vi "FindAllSupportedModules.vi"(11 "Device Model":T1) -> (2 "All Supported Modules":string[](array[string]), 3 "Number of Supported Modules":i32)   [LabVIEW 2015]
uses:
  <vilib>/addons/InsightCM/MessageBus/Base/controls/Device.ctl
  <vilib>/addons/InsightCM/MessageBus/Base/controls/KeyValuePair.ctl
  <vilib>/addons/InsightCM/MessageBus/Base/controls/DataGroup.ctl
  <vilib>/addons/InsightCM/MessageBus/Base/controls/OperatingState.ctl
  <vilib>/addons/InsightCM/MessageBus/Base/controls/Trigger.ctl
  <vilib>/addons/InsightCM/MessageBus/Base/controls/Condition.ctl
  <vilib>/addons/InsightCM/Utilities/DeviceModelHelpers/DeviceModelHelpers.lvlib
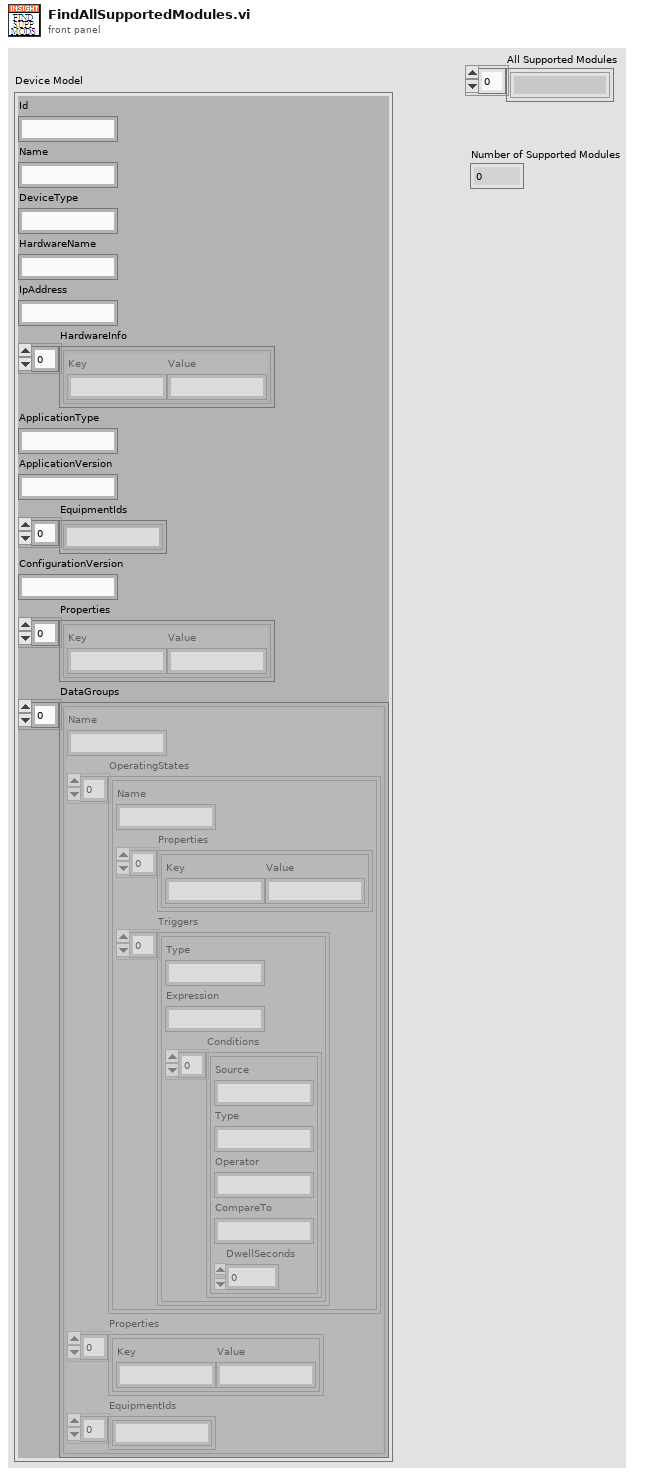
[diagram p1: front panel]
types:
  T1 = typedef "Device.ctl" = cluster{"Id":string, "Name":string, "DeviceType":string, "HardwareName":string, "IpAddress":string, "HardwareInfo":T2[], "ApplicationType":string, "ApplicationVersion":string, "EquipmentIds":string[], "ConfigurationVersion":string, "Properties":T2[], "DataGroups":T3[]}
  T2 = typedef "KeyValuePair.ctl" = cluster{"Key":string, "Value":string}
  T3 = typedef "DataGroup.ctl" = cluster{"Name":string, "OperatingStates":T4[], "Properties":T2[], "EquipmentIds":string[]}
  T4 = typedef "OperatingState.ctl" = cluster{"Name":string, "Properties":T2[], "Triggers":T5[]}
  T5 = typedef "Trigger.ctl" = cluster{"Type":string, "Expression":string, "Conditions":T6[]}
  T6 = typedef "Condition.ctl" = cluster{"Source":string, "Type":string, "Operator":string, "CompareTo":string, "DwellSeconds":dbl}
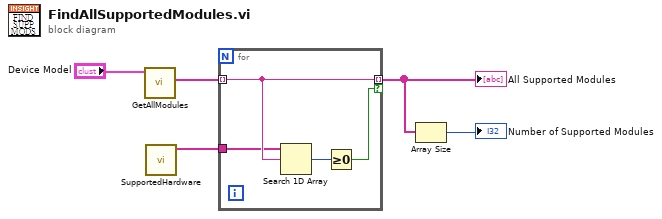
[diagram p0: block diagram]
diagram:
  n1 = call <vilib>:"GetAllModules.vi"("device in"="Device Model") -> ("all modules"=w4:string[])  [unwired: 9 in, 1 out]
  n2 = call "SupportedHardware.vi"() -> ("Supported Hardware"=w1:string[])  [unwired: 11 in]
  n3 = for {
    tunnel: w4 -> [w8] mode=indexing
    tunnel: [w8] -> w3 mode=indexing if=w7
    tunnel: w1 -> [w6]
    n4 = Search 1D Array(1D array=w6, element=w8) -> (index of element=w9:i32)  [unwired: 1 in]
    n5 = Greater Or Equal To 0?(x=w9) -> (x >= 0?=w7:bool)
  }
  "All Supported Modules" <- w3
  n6 = Array Size(array=w3) -> (size(s)=→"Number of Supported Modules":i32)
